vi "test-json-schema-recursive-defs.vi"() -> ()   [LabVIEW 2019, in "TEST-JSON-Schema.lvlib"]
uses:
  TEST-JSON-Schema.lvlib
  typedefs/test_enum--enum.ctl
  typedefs/test_cluster--cluster.ctl
  typedefs/test_nested_cluster--cluster.ctl
  JSON-Schema/JSON-Schema.lvlib
  <vilib>/JDP Science/JSONtext/JSONtext.lvlib
  <vilib>/Utility/Data Type/NI_Data Type.lvlib
panel:
  out "Array":string[](array[string])
  out "JSON Schema":string
  out "Array 2":bool[](array[boolean])
  out "JSON Schema out":string
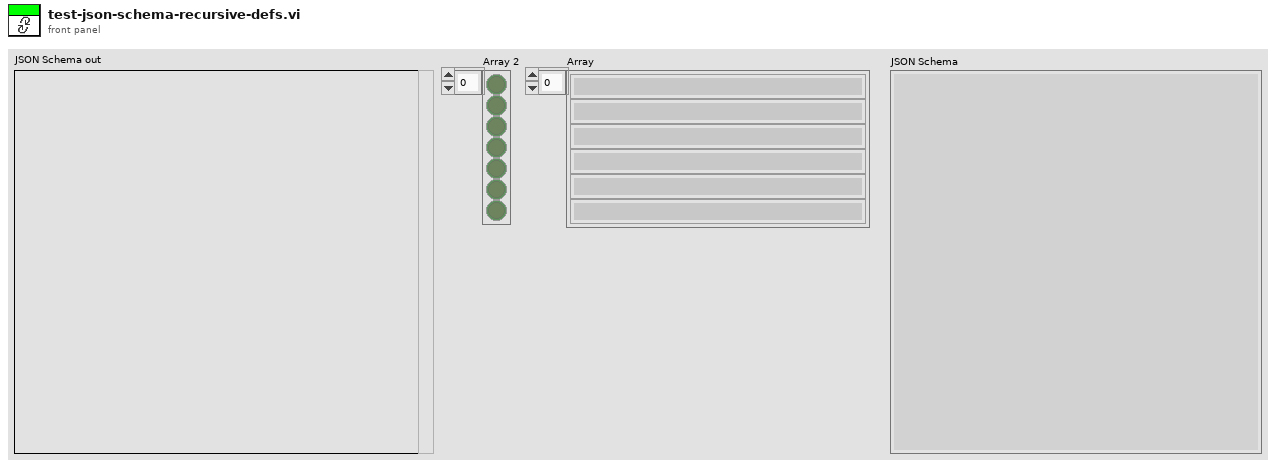
[diagram p1: front panel]
types:
  T1 = typedef "TEST-JSON-Schema.lvlib/test_nested_cluster--cluster.ctl" = cluster{"string":string, "test_cluster":T2}
  T2 = typedef "TEST-JSON-Schema.lvlib/test_cluster--cluster.ctl" = cluster{"numeric":dbl, "test_enum":T3}
  T3 = typedef "TEST-JSON-Schema.lvlib/test_enum--enum.ctl" = enum16{"option_1", "option_2"}
  T4 = enum32{"Bad", "Idle", "Run top level", "Running"}
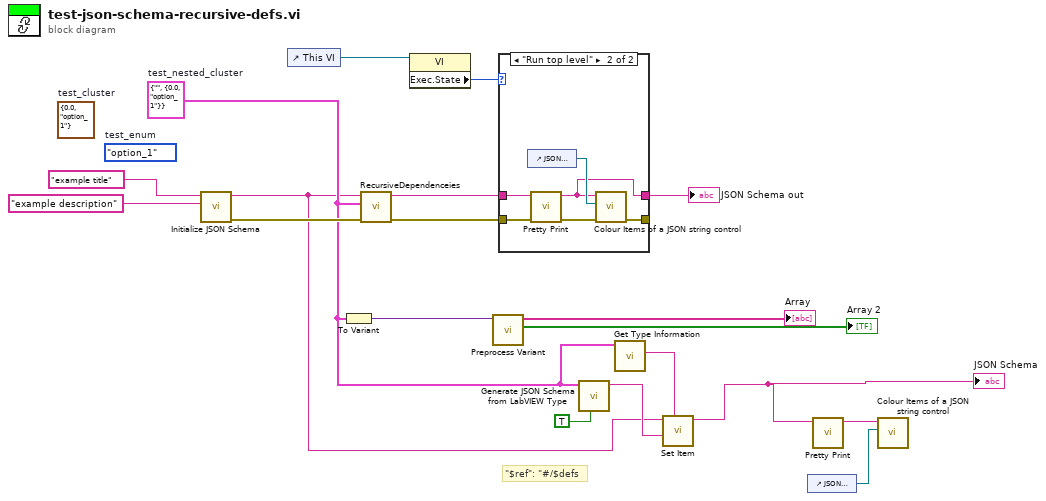
[diagram p0: block diagram]
diagram:
  w4 = T1 {"string"="", "test_cluster"={"numeric"=0.0, "test_enum"=enum."option_1"}}  # test_nested_cluster
  (unwired) T2 {"numeric"=0.0, "test_enum"=enum."option_1"}  # test_cluster
  (unwired) test_enum--enum."option_1"  # test_enum
  # "\"$ref\": \"#/$defs"
  n1 = call "Initialize JSON Schema.vi"("Description"="example description", "Title"="example title") -> ("error out"=w14:errorcluster, "JSON Schema out"=w1:string)  [unwired: 8 in]
  n2 = control-ref of="This VI"() -> (w19:refnum<vi>)
  n3 = To Variant(anything=w4) -> (Variant=w6:variant)
  n4 = call "RecursiveDependenceies.vi"("error in (no error)"=w14, "Object"=w4, "JSON Schema in"=w1) -> ("error out"=w12:errorcluster, "JSON Schema out"=w13:string)  [unwired: 7 in]
  n5 = property class="VI"(reference=w19) -> ("Exec.State"=w18:T4)  [unwired: 1 in, 2 out]
  n6 = call "Preprocess Variant.vi"("Variant"=w6) -> ("Array"=→"Array 2":bool[], "Array 2"=→"Array":string[])  [unwired: 9 in]
  n7 = case shown="\"Run top level\"" w18 {
    tunnel: w13 -> [w20 w27]
    tunnel: w12 -> [w21 w26]
    tunnel: [w21 w24] -> _
    tunnel: [w20 w22] -> w17
    frame Default {
    }
    frame "Run top level" {
      n8 = control-ref of="JSON Schema out"() -> (w23:refnum<vi>)
      n9 = call <vilib>:"Pretty Print.vi"("error in (no error)"=w26, "JSON"=w27) -> ("error out"=w25:errorcluster, "<JSON>"=w22:string)  [unwired: 7 in, 1 out]
      n10 = call <vilib>:"Colour Items of a JSON string control.vi"("error in (no error)"=w25, "String Control"=w23, "JSON"=w22) -> ("error out"=w24:errorcluster)  [unwired: 8 in]
    }
  }
  "JSON Schema out" <- w17
  n11 = call <vilib>:"Generate JSON Schema from LabVIEW Type.vi"("Strict Clusters"=TRUE, "Variant"=w4) -> ("JSON Schema"=w3:string)  [unwired: 8 in, 1 out]
  n12 = call <vilib>:"Get Type Information.vi"("variant"=w4) -> ("name"=w5:string)  [unwired: 6 in, 4 out]
  n13 = call <vilib>:"Set Item.vi"("$Path or Item Name"=w5, "JSON to Insert"=w3, "JSON"=w1) -> ("<JSON>"=w2:string)  [unwired: 5 in, 2 out]
  "JSON Schema" <- w2
  n14 = control-ref of="JSON Schema"() -> (w7:refnum<vi>)
  n15 = call <vilib>:"Pretty Print.vi"("JSON"=w2) -> ("<JSON>"=w8:string)  [unwired: 8 in, 2 out]
  n16 = call <vilib>:"Colour Items of a JSON string control.vi"("String Control"=w7, "JSON"=w8) -> ()  [unwired: 9 in, 1 out]
